vi "IPS Read Magnet Current.vi"(3 "Error In":errorcluster={"status"=FALSE, "code"=1073676294, "source"="VISA Read in Prologix USB GPIB Command.vi"}, 5 "VISA resource name":refnum<visa-resource-name>="COM3") -> (0 "Error Out":errorcluster={"status"=FALSE, "code"=1073676294, "source"="VISA Read in Prologix_GPIB_Sample.vi"}, 1 "Magnet Current (A)":dbl, 2 "VISA resource name":refnum<visa-resource-name>="GPIB1::25::INSTR")   [LabVIEW 2013]
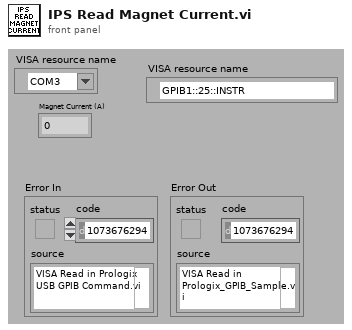
[diagram p1: front panel]
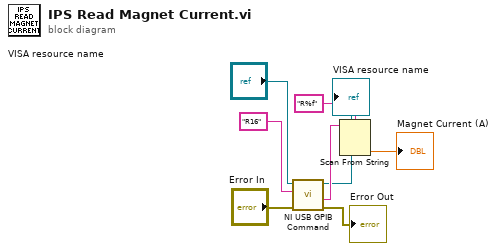
[diagram p0: block diagram]
diagram:
  n1 = call "NI USB GPIB Command.vi"("Error In"="Error In", "String to Send"="R16", "VISA resource name"="VISA resource name") -> ("Error Out"=→"Error Out":errorcluster, "Return String from Device (Not all commands return a String)"=w3:string, "VISA resource name"=→"VISA resource name":refnum<visa-resource-name>)  [unwired: 1 in, 1 out]
  n2 = Scan From String(format string="R%f", input string=w3) -> (output 1=→"Magnet Current (A)":dbl)  [unwired: 2 in, 4 out]
